vi "Refresh Panel Instruments.vi"(8 "error in":errorcluster, 11 "Instruments in":refnum<class "Instruments.lvclass">) -> (0 "error out":errorcluster, 3 "Instruments out":refnum<class "Instruments.lvclass">)   [LabVIEW 2023, in "Instruments.lvlib" / "Instruments.lvclass"]
doc: "Use instrument name to find self reference in list of panel referenes."
uses:
  Library/Instruments.lvclass
  C:/Users/Public/Documents/Development/builds/Engine/Actor Framework.lvlibp/1abvi3w/vi.lib/ActorFramework/Actor/Actor.lvclass
  Library/Instruments.lvclass/Instruments.ctl
  builds/Engine/Actor Framework.lvlibp/1abvi3w/vi.lib/ActorFramework/Actor/Read Actor Label.vi
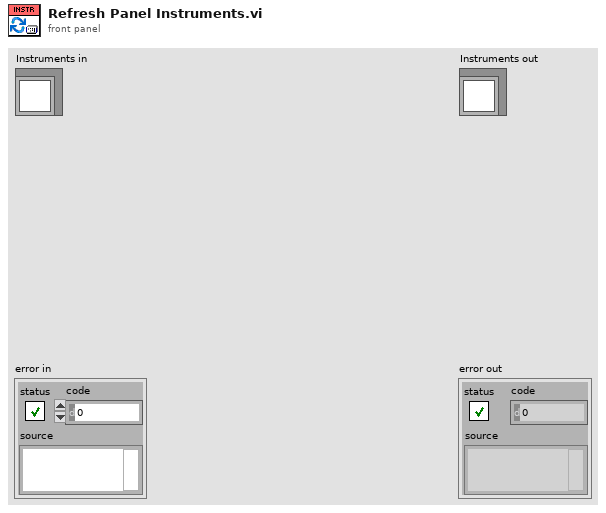
[diagram p1: front panel]
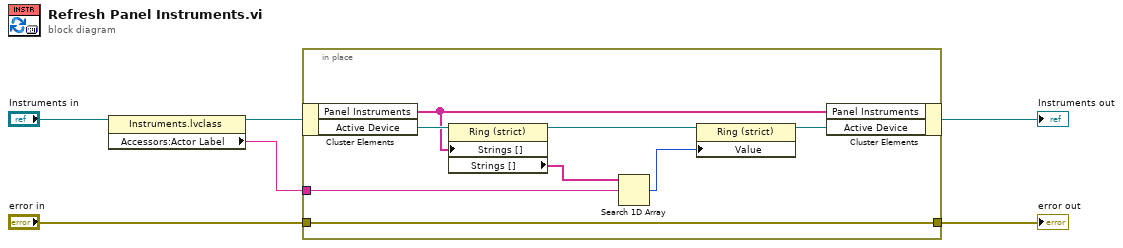
[diagram p0: block diagram]
diagram:
  n1 = property class="Instruments.lvclass"(reference="Instruments in") -> (reference out=w2:refnum<class "Instruments.lvclass">, "Accessors:Actor Label"=w1:string)  [unwired: 1 in, 1 out]
  n2 = in-place {
    in-place-border: "error in" -> [w10]
    in-place-border: [w10] -> w5
    in-place-border: w1 -> [w9]
    n3 = in-place-cluster #1(w2) -> ("Panel Instruments"=w7:string[], "Active Device"=w14:refnum<vi>)
    n4 = property class="Ring (strict)"(reference=w14, "Strings []"=w7) -> (reference out=w13:refnum<vi>, "Strings []"=w8:string[])  [unwired: 1 in, 1 out]
    n5 = Search 1D Array(1D array=w8, element=w9) -> (index of element=w11:i32)  [unwired: 1 in]
    n6 = property class="Ring (strict)"(reference=w13, "Value"=w11) -> (reference out=w12:refnum<vi>)  [unwired: 1 in, 1 out]
    n7 = in-place-cluster #1("Panel Instruments"=w7, "Active Device"=w12) -> (→"Instruments out":refnum<class "Instruments.lvclass">)
  }
  "error out" <- w5
